vi "Symphony GetMaxVal.vi"(6 "PixelArr":dbl[](array[numeric]), 8 "error in (no error)":errorcluster caption="entrée d'erreur (pas d'erreur)", 10 "MaxFind":T1, 11 "DataArr":dbl[](array[numeric])) -> (0 "error out":errorcluster caption="sortie d'erreur", 2 "Max_and_Pix":dbl[](array[numeric]))   [LabVIEW 2019]
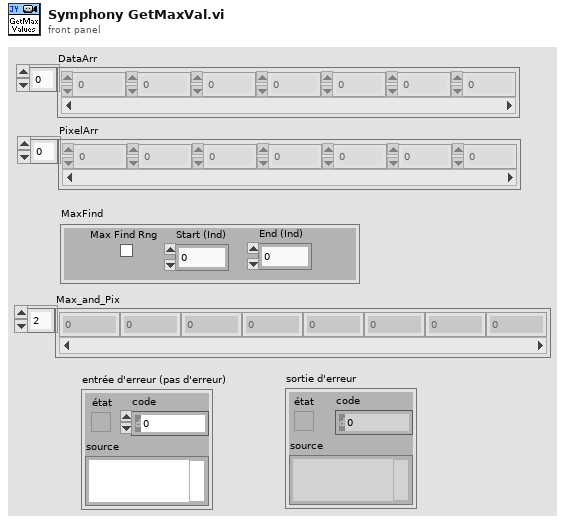
[diagram p1: front panel]
types:
  T1 = cluster{"Max Find Rng":bool, "MaxFindStart":i32, "MaxFindEnd":i32}
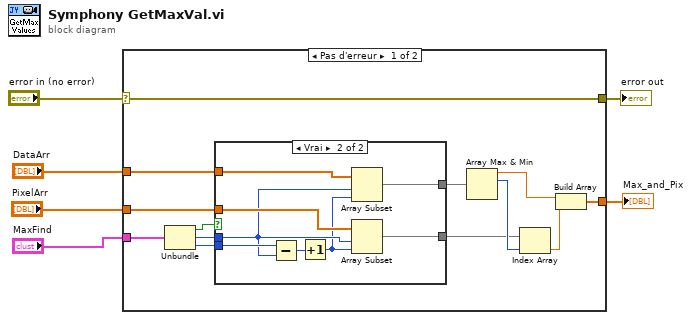
[diagram p0: block diagram]
diagram:
  n1 = case shown="Pas d'erreur" "error in (no error)" {
    selector: "error in (no error)" -> [w7 w30]
    tunnel: [w7 w30] -> w6
    tunnel: "PixelArr" -> [w17 _]
    tunnel: "MaxFind" -> [w18 _]
    tunnel: "DataArr" -> [w13 _]
    tunnel: [w8 _] -> w1
    frame No Error {
      n2 = Unbundle(w18) -> ("Max Find Rng"=w15:bool, "MaxFindStart"=w16:i32, "MaxFindEnd"=w19:i32)
      n3 = case shown="Vrai" w15 {
        tunnel: w19 -> [_ w28]
        tunnel: w17 -> [w20 w27]
        tunnel: w16 -> [_ w25]
        tunnel: w13 -> [w21 w26]
        tunnel: [w21 w23] -> w11
        tunnel: [w20 w22] -> w12
        frame False {
        }
        frame True {
          n4 = Subtract(x=w28, y=w25) -> (x-y=w29:i32)
          n5 = Increment(x=w29) -> (x+1=w24:i32)
          n6 = Array Subset(array=w26, index=w25, length=w24) -> (w23:dbl[])
          n7 = Array Subset(array=w27, index=w25, length=w24) -> (w22:dbl[])
        }
      }
      n8 = Array Max & Min(array=w11) -> (max value=w10:dbl, max index (indices)=w14:i32)  [unwired: 2 out]
      n9 = Index Array(array=w12, index=w14) -> (element=w9:dbl)
      n10 = Build Array(w10, w9) -> (w8:dbl[])
    }
    frame Error {
    }
  }
  "error out" <- w6
  "Max_and_Pix" <- w1
